vi "Graph_cluster.vi"() -> ()   [LabVIEW 2016]
panel:
  in  "Array 3":dbl[](array[numeric])=[0.0, 4.0, 5.0, 8.0, 4.0, 0.0, 5.0, 9.0, 10.0, 9.0]
  in  "Array 2":dbl[](array[numeric])=[0.0, 4.0, 5.0, 8.0, 4.0, 0.0, 5.0, 9.0, 10.0, 9.0]
  in  "Array":dbl[](array[numeric])=[0.0, 4.0, 5.0, 8.0, 4.0, 0.0, 5.0, 9.0, 10.0, 9.0]
  out "Waveform Graph":cluster{"X0":dbl, "X":dbl, "Array":dbl[]}(graph)
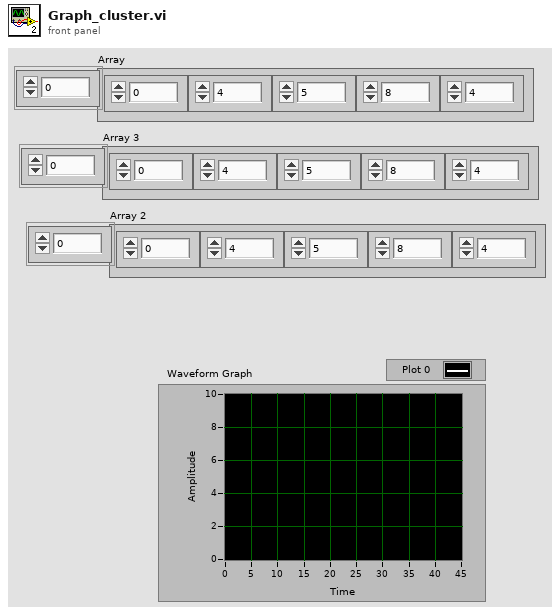
[diagram p1: front panel]
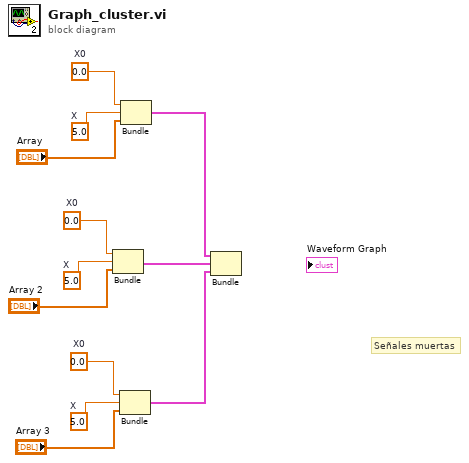
[diagram p0: block diagram]
diagram:
  w5 = 5.0  # X
  w6 = 0.0  # X0
  w8 = 5.0  # X
  w9 = 0.0  # X0
  w11 = 5.0  # X
  w12 = 0.0  # X0
  # "Señales muertas"
  n1 = Bundle("X0"=w9, "X"=w8, "Array 2"="Array 2") -> (w3:cluster{"X0":dbl, "X":dbl, "Array 2":dbl[]})  [unwired: 1 in]
  n2 = Bundle("X0"=w6, "X"=w5, "Array 3"="Array 3") -> (w1:cluster{"X0":dbl, "X":dbl, "Array 3":dbl[]})  [unwired: 1 in]
  n3 = Bundle("X0"=w12, "X"=w11, "Array"="Array") -> (w2:cluster{"X0":dbl, "X":dbl, "Array":dbl[]})  [unwired: 1 in]
  n4 = Bundle(w2, w3, w1) -> ()  [unwired: 1 in, 1 out]
